vi "LPD_Remove All Whitespace.vi"(2 "String":string) -> (7 "String out":string)   [LabVIEW 2009]
doc: "Removes all white space from a string.\nWhitespace is a character such as Space, Tab, Newline, Carriage Return, Form Feed, or Vertical Tab.\n\n\nAuthor: Mike Schultz\n\n\nLogicPD, Inc\nwww.logicpd.com"
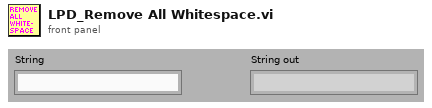
[diagram p1: front panel]
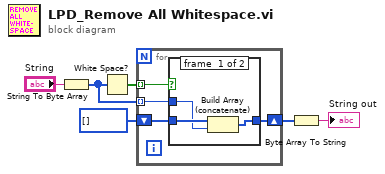
[diagram p0: block diagram]
diagram:
  n1 = String To Byte Array(string="String") -> (unsigned byte array=w4:u8[])
  n2 = White Space?(1:w4) -> (0:w5:bool[])
  n3 = for {
    tunnel: w5 -> [w10] mode=indexing
    tunnel: w4 -> [w7] mode=indexing
    shift-right: [w9] -> w3
    shift-left: u8[] [] -> [w8]
    n4 = case shown="False" w10 {
      tunnel: [w13 w14] -> w9
      tunnel: w8 -> [w12 w14]
      tunnel: w7 -> [w11 _]
      frame #0 {
        n5 = Build Array (concatenate)(w12, w11) -> (w13:u8[])
      }
      frame #1 {
        # "White Space"
      }
    }
  }
  n6 = Byte Array To String(unsigned byte array=w3) -> (string=→"String out":string)
